vi "TimerWithoutDAQmxSubvi.vi"(9 "Condition":dbl=162.0, 10 "Period (Sec)":dbl=182.0 format="%#_13g", 11 "milliseconds to wait":u32=100) -> ()   [LabVIEW 2018]
panel:
  out "PulseNumber Now":dbl=10.0
  out "Pulse Number":dbl=10.0
  out "Waveform Chart":i32(graph)
  out "floor(x/y) 2":i32=1
  out "floor(x/y)":dbl=39.0
  out "x >= y?":bool
  out "Numeric":i32=221
  in  "stop 3":bool
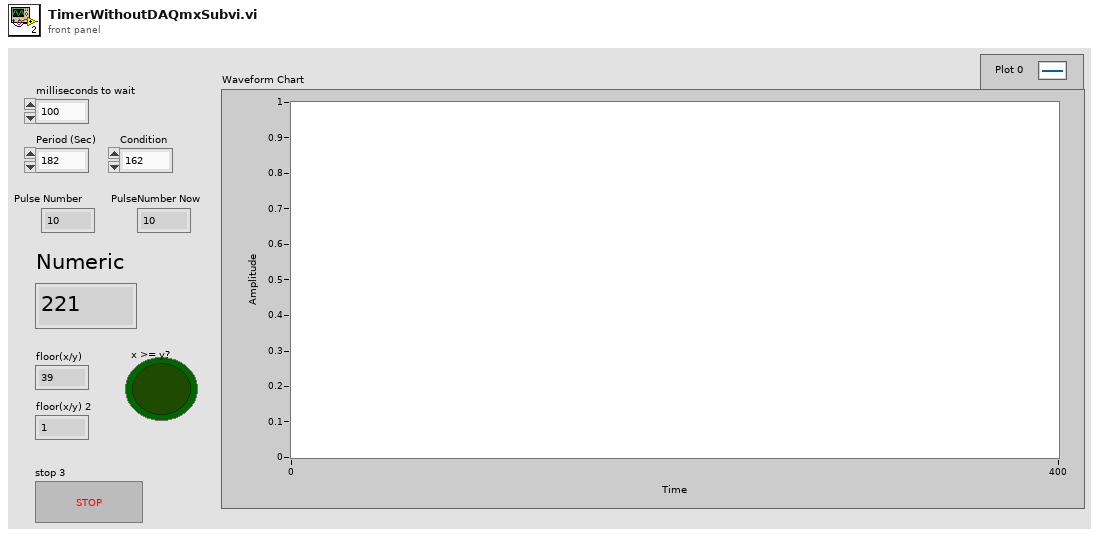
[diagram p1: front panel]
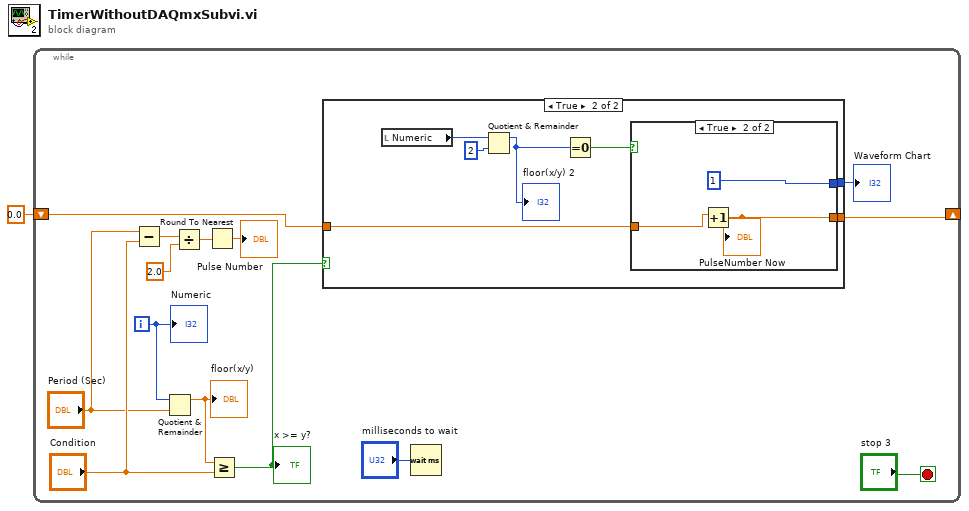
[diagram p0: block diagram]
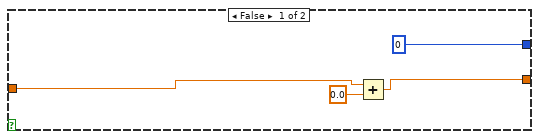
[diagram p2: hidden frame]
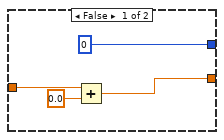
[diagram p3: hidden frame]
diagram:
  n1 = while {
    shift-right: [w3] -> _
    shift-left: 0.0 -> [w2]
    i -> [w13]
    stop <- "stop 3" stop-if-true
    n2 = Subtract(x="Period (Sec)", y="Condition") -> (x-y=w8:dbl)
    n3 = Quotient & Remainder(x=w13, y="Period (Sec)") -> (x-y*floor(x/y)=w12:dbl)  [unwired: 1 out]
    "floor(x/y)" <- w12
    n4 = Divide(x=w8, y=2.0) -> (x/y=w6:dbl)
    n5 = Round To Nearest(number=w6) -> (nearest integer value=→"Pulse Number":dbl)
    n6 = Greater Or Equal?(x=w12, y="Condition") -> (x >= y?=w11:bool)
    "x >= y?" <- w11
    n7 = case shown="True" w11 {
      tunnel: [0 w22] -> w10
      tunnel: [w16 w21] -> w3
      tunnel: w2 -> [w17 w20]
      frame False {
        n8 = Add(x=w17, y=0.0) -> (x+y=w16:dbl)
      }
      frame True {
        n9 = local read "Numeric"() -> (w26:i32)
        n10 = Quotient & Remainder(x=w26, y=2) -> (x-y*floor(x/y)=w23:i32)  [unwired: 1 out]
        "floor(x/y) 2" <- w23
        n11 = Equal To 0?(x=w23) -> (x = 0?=w25:bool)
        n12 = case shown="True" w25 {
          tunnel: [0 1] -> w22
          tunnel: [w27 w32] -> w21
          tunnel: w20 -> [w29 w31]
          frame False {
            n13 = Add(x=w29, y=0.0) -> (x+y=w27:dbl)
          }
          frame True {
            n14 = Increment(x=w31) -> (x+1=w32:dbl)
            "PulseNumber Now" <- w32
          }
        }
      }
    }
    "Waveform Chart" <- w10
    n15 = Wait (ms)(milliseconds to wait="milliseconds to wait") -> ()  [unwired: 1 out]
    "Numeric" <- w13
  }
